vi "read_As_liq0.vi"() -> (3 "Actual As liq Flow Rate":dbl, 4 "As liq Remote":bool, 5 "As liq Run":bool, 6 "As liq Bubbler":bool, 7 "As liq Active":bool)   [LabVIEW 2011]
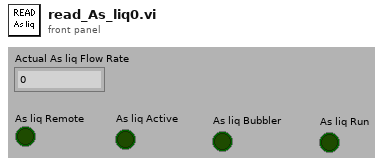
[diagram p1: front panel]
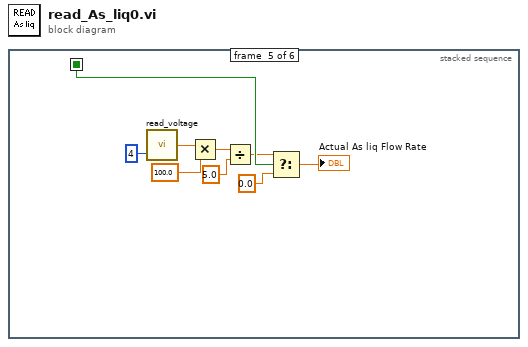
[diagram p0: block diagram]
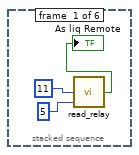
[diagram p2: hidden frame]
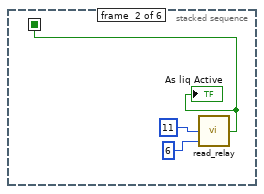
[diagram p3: hidden frame]
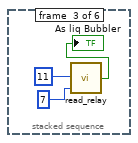
[diagram p4: hidden frame]
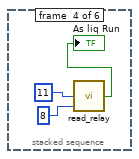
[diagram p5: hidden frame]
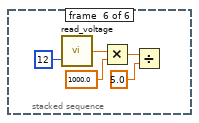
[diagram p6: hidden frame]
diagram:
  n1 = stacked-sequence {
    seq-local: [_ w4 _ _ _ _] -> [_ _ _ _ w16 _]
    frame #0 {
      n2 = call "read_relay.vi"("Relay"=5, "Slot"=11) -> ("Relay Status"=→"As liq Remote":bool)  [unwired: 1 out]
    }
    frame #1 {
      n3 = call "read_relay.vi"("Relay"=6, "Slot"=11) -> ("Relay Status"=w4:bool)  [unwired: 1 out]
      "As liq Active" <- w4
    }
    frame #2 {
      n4 = call "read_relay.vi"("Relay"=7, "Slot"=11) -> ("Relay Status"=→"As liq Bubbler":bool)  [unwired: 1 out]
    }
    frame #3 {
      n5 = call "read_relay.vi"("Relay"=8, "Slot"=11) -> ("Relay Status"=→"As liq Run":bool)  [unwired: 1 out]
    }
    frame #4 {
      n6 = call "read_voltage.vi"("Channel"=4) -> ("Voltage"=w20:dbl)  [unwired: 1 in]
      n7 = Multiply(x=w20, y=100.0) -> (x*y=w18:dbl)
      n8 = Divide(x=w18, y=5.0) -> (x/y=w15:dbl)
      n9 = Select(t=w15, s=w16, f=0.0) -> (s? t:f=→"Actual As liq Flow Rate":dbl)
    }
    frame #5 {
      n10 = call "read_voltage.vi"("Channel"=12) -> ("Voltage"=w25:dbl)  [unwired: 1 in]
      n11 = Multiply(x=w25, y=1000.0) -> (x*y=w23:dbl)
      n12 = Divide(x=w23, y=5.0) -> ()  [unwired: 1 out]
    }
  }
